vi "CalcGateTiming.vi"(11 "Bouncer Settings":T1) -> (1 "low time":dbl, 4 "High time":dbl)   [LabVIEW 2011]
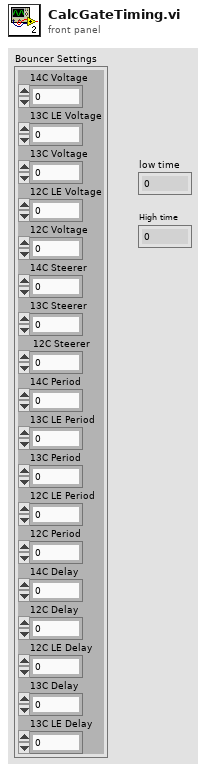
[diagram p1: front panel]
types:
  T1 = cluster{"14C Voltage":dbl, "13C LE Voltage":dbl, "13C Voltage":dbl, "12C LE Voltage":dbl, "12C Voltage":dbl, "14C Steerer":dbl, "13C Steerer":dbl, " 12C Steerer":dbl, "14C Period":dbl, "13C LE Period":dbl, "13C Period":dbl, "12C LE Period":dbl, "12C Period":dbl, "14C Delay":dbl, "12C Delay":dbl, "12C LE Delay":dbl, "13C Delay":dbl, "13C LE Delay":dbl}
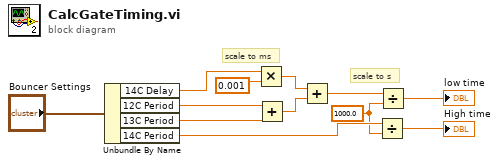
[diagram p0: block diagram]
diagram:
  w4 = 1000.0 ("y")
  # "scale to s"
  # "scale to ms"
  n1 = Unbundle By Name("Bouncer Settings") -> ("14C Delay"=w2:dbl, "12C Period"=w10:dbl, "13C Period"=w11:dbl, "14C Period"=w12:dbl)
  n2 = Multiply(x=w2, y=0.001) -> (x*y=w9:dbl)
  n3 = Add(x=w10, y=w11) -> (x+y=w5:dbl)
  n4 = Add(x=w9, y=w5) -> (x+y=w3:dbl)
  n5 = Divide(x=w12, y=w4) -> (x/y=→"High time":dbl)
  n6 = Divide(x=w3, y=w4) -> (x/y=→"low time":dbl)
